vi "UsrProfiles-Read changes from FGVs.vi"(11 "error in (no error)":errorcluster) -> (3 "All changed parameters info":T7[](array[typedef]), 4 "Changes exist":bool, 6 "Keys of changed parameters-DBL":T5, 8 "Keys of changed parameters-STRING":T1, 10 "Keys of changed parameters-BOOL":T3, 15 "error out":errorcluster)   [LabVIEW 2013]
uses:
  Typedefs/Changed parameter cluster.ctl
  Typedefs/Changes info cluster-DBL.ctl
  Configuration code/Typedefs/Ini file interface (DBL).ctl
  Typedefs/Changes info cluster-BOOL.ctl
  Configuration code/Typedefs/Ini file interface (Boolean).ctl
  Typedefs/Changes info cluster-STRING.ctl
  Configuration code/Typedefs/Ini file interface (String).ctl
  Typedefs/Comparison states.ctl
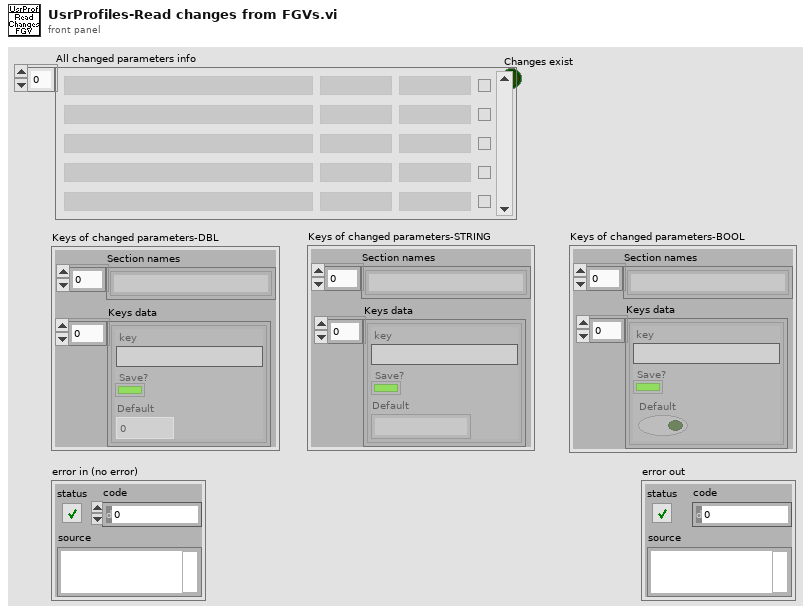
[diagram p1: front panel]
types:
  T1 = typedef "Changes info cluster-STRING.ctl" = cluster{"Section names":string[], "Keys data":T2}
  T2 = typedef "Ini file interface (String).ctl" = cluster{"key":string, "Save?":bool, "Default":string}[]
  T3 = typedef "Changes info cluster-BOOL.ctl" = cluster{"Section names":string[], "Keys data":T4}
  T4 = typedef "Ini file interface (Boolean).ctl" = cluster{"key":string, "Save?":bool, "Default":bool}[]
  T5 = typedef "Changes info cluster-DBL.ctl" = cluster{"Section names":string[], "Keys data":T6}
  T6 = typedef "Ini file interface (DBL).ctl" = cluster{"key":string, "Save?":bool, "Default":dbl}[]
  T7 = typedef "Changed parameter cluster.ctl" = cluster{"Name":string, "Old value":string, "New value":string, "Save":bool}
  T8 = typedef "Comparison states.ctl" = enum16{"Init.", "Add", "Read"}
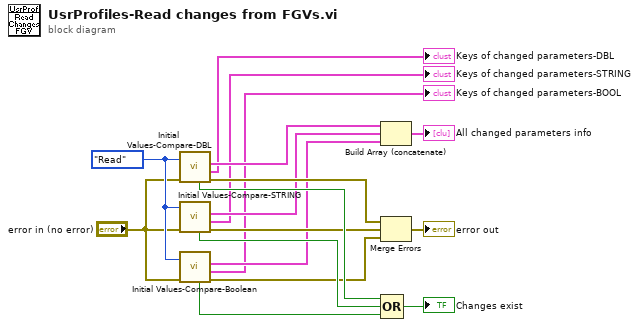
[diagram p0: block diagram]
diagram:
  w17 = Comparison_states."Read" ("Function (Add)")
  n1 = call "Initial Values-Compare-DBL.vi"("Function (Add)"=w17, "error in (no error)"="error in (no error)") -> ("error out"=w9:errorcluster, "Output info"=→"Keys of changed parameters-DBL":T5, "Changed parameters info"=w7:T7[], "Changes exist"=w13:bool)  [unwired: 5 in, 1 out]
  n2 = call "Initial Values-Compare-STRING.vi"("Function (Add)"=w17, "error in (no error)"="error in (no error)") -> ("error out"=w10:errorcluster, "Keys of changed parameters"=→"Keys of changed parameters-STRING":T1, "Changed parameters info"=w6:T7[], "Changes exist"=w14:bool)  [unwired: 5 in, 1 out]
  n3 = call "Initial Values-Compare-Boolean.vi"("Function (Add)"=w17, "error in (no error)"="error in (no error)") -> ("error out"=w11:errorcluster, "Keys of changed parameters"=→"Keys of changed parameters-BOOL":T3, "Changed parameters info"=w5:T7[], "Changes exist"=w16:bool)  [unwired: 5 in, 1 out]
  n4 = Build Array (concatenate)(w7, w6, w5) -> (→"All changed parameters info":T7[])
  n5 = Merge Errors(w9, w10, w11) -> (→"error out":errorcluster)
  n6 = Compound Arithmetic op=OR(w13, w14, w16) -> (→"Changes exist":bool)
